vi "LCDPrint.vi"(8 "error in (no error)":errorcluster, 10 "TextToWrite":string, 11 "LCDRef":T1) -> (0 "error out":errorcluster)   [LabVIEW 2013]
uses:
  LCDRef.ctl
  <vilib>/Rock Robotics/WPI/SerialPort/WPI_SerialPortRef.ctl
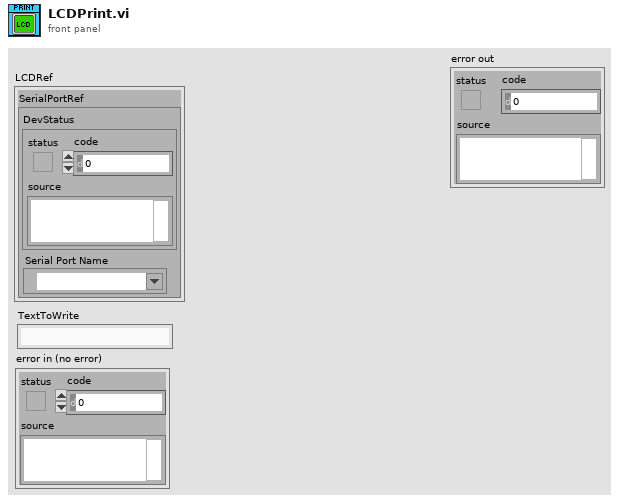
[diagram p1: front panel]
types:
  T1 = typedef "LCDRef.ctl" = cluster{"SerialPortRef":T2}
  T2 = typedef "WPI_SerialPortRef.ctl" = cluster{"DevStatus":errorcluster, "Serial Port Name":refnum<visa-resource-name>}
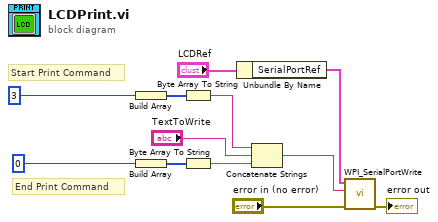
[diagram p0: block diagram]
diagram:
  # "End Print Command"
  # "Start Print Command"
  n1 = Build Array(u8 3 ("element")) -> (w9:u8[])
  n2 = Build Array(u8 0 ("element")) -> (w7:u8[])
  n3 = Byte Array To String(unsigned byte array=w9) -> (string=w6:string)
  n4 = Byte Array To String(unsigned byte array=w7) -> (string=w4:string)
  n5 = Unbundle By Name("LCDRef") -> ("SerialPortRef"=w12:T2)
  n6 = Concatenate Strings(w6, "TextToWrite", w4) -> (w3:string)
  n7 = call <vilib>:"WPI_SerialPortWrite.vi"("error in (no error)"="error in (no error)", "Buffer"=w3, "SerialPortRef"=w12) -> ("error out"=→"error out":errorcluster)  [unwired: 6 in, 2 out]
